vi "petWatchdog.vi"(10 "RT Safe":bool, 11 "FPGA VI Reference In":refnum<k20>) -> (3 "FPGA VI Reference Out":refnum<k20>)   [LabVIEW 2017]
uses:
  <vilib>/Utility/error.llb/Error Cluster From Error Code.vi
  <vilib>/rvi/errors/niLvFpgaAdjustHostInterfaceError.vi
  <vilib>/rvi/interface/nirviReadWriteControl/nirviReadWriteControl.xnode
  RT Watchdog.lvlib
  NiFpgaLv.dll
  <vilib>/rvi/interface/Simulation/niFpgaSimulationCallBeginRW.vi
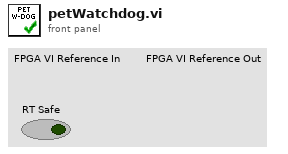
[diagram p1: front panel]
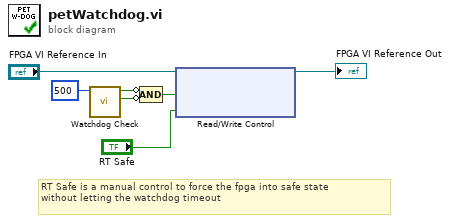
[diagram p0: block diagram]
diagram:
  # "RT Safe is a manual control to force the fpga into safe state\nwithout letting the watchdog timeout"
  n1 = call "Watchdog Check.vi"("Timeout (ms)"=u32 500) -> ("Skipped?"=w7:bool, "Timeout?"=w6:bool)  [unwired: 8 in, 1 out]
  n2 = Compound Arithmetic op=AND(invert w6, invert w7) -> (w3:bool)
  n3 = xnode "Read/Write Control"("FPGA VI Reference In"="FPGA VI Reference In", "Pet RT Watchdog"=w3, "RT Safe"="RT Safe") -> ("FPGA VI Reference Out"=→"FPGA VI Reference Out":refnum<k20>)  [unwired: 1 in, 1 out]
